vi "Zamojski_10_sub_1.vi"(8 "error in (no error)":errorcluster) -> (0 "error out":errorcluster)   [LabVIEW 2020]
uses:
  <vilib>/measure/NI_MABase.lvlib
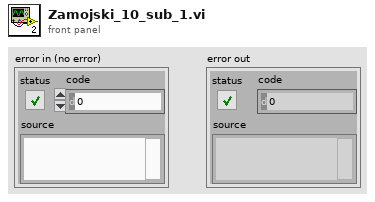
[diagram p1: front panel]
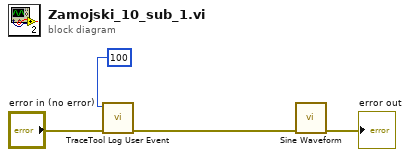
[diagram p0: block diagram]
diagram:
  n1 = call <vilib>:"TraceTool Log User Event.vi"("error in (no error)"="error in (no error)", "Event ID (0-255)"=u32 100) -> ("error out"=w3:errorcluster)  [unwired: 9 in]
  n2 = call <vilib>:"Sine Waveform.vi"("error in (no error)"=w3) -> ("error out"=→"error out":errorcluster)  [unwired: 9 in, 1 out]
